vi "Intialise or refresh queue.vi"(2 "When did you stick it in?":dbl, 3 "Cell Settings Array":T3=[{"Measure?"=TRUE, "Area (cm^2)"=0.0, "Cell Label"="", "Cell Description"="", "Time between scans (s)"=0.0, "Cell Position"=1, "Scan settings in queue"=0, "Sample holder"=4.0, "User name"=""}, {"Measure?"=TRUE, "Area (cm^2)"=0.0, "Cell Label"="", "Cell Description"="", "Time between scans (s)"=0.0, "Cell Position"=2, "Scan settings in queue"=0, "Sample holder"=4.0, "User name"=""}, {"Measure?"=TRUE, "Area (cm^2)"=0.0, "Cell Label"="", "Cell Description"="", "Time between scans (s)"=0.0, "Cell Position"=3, "Scan settings in queue"=0, "Sample holder"=4.0, "User name"=""}, {"Measure?"=TRUE, "Area (cm^2)"=0.0, "Cell Label"="", "Cell Description"="", "Time between scans (s)"=0.0, "Cell Position"=4, "Scan settings in queue"=0, "Sample holder"=4.0, "User name"=""}, {"Measure?"=TRUE, "Area (cm^2)"=0.0, "Cell Label"="", "Cell Description"="", "Time between scans (s)"=0.0, "Cell Position"=5, "Scan settings in queue"=0, "Sample holder"=4.0, "User name"=""}, {"Measure?"=TRUE, "Area (cm^2)"=0.0, "Cell Label"="", "Cell Description"="", "Time between scans (s)"=0.0, "Cell Position"=6, "Scan settings in queue"=0, "Sample holder"=4.0, "User name"=""}, {"Measure?"=TRUE, "Area (cm^2)"=0.0, "Cell Label"="", "Cell Description"="", "Time between scans (s)"=0.0, "Cell Position"=7, "Scan settings in queue"=0, "Sample holder"=4.0, "User name"=""}, {"Measure?"=TRUE, "Area (cm^2)"=0.0, "Cell Label"="", "Cell Description"="", "Time between scans (s)"=0.0, "Cell Position"=8, "Scan settings in queue"=0, "Sample holder"=4.0, "User name"=""}, {"Measure?"=TRUE, "Area (cm^2)"=0.0, "Cell Label"="", "Cell Description"="", "Time between scans (s)"=0.0, "Cell Position"=9, "Scan settings in queue"=0, "Sample holder"=4.0, "User name"=""}, {"Measure?"=TRUE, "Area (cm^2)"=0.0, "Cell Label"="", "Cell Description"="", "Time between scans (s)"=0.0, "Cell Position"=10, "Scan settings in queue"=0, "Sample holder"=4.0, "User name"=""}, {"Measure?"=TRUE, "Area (cm^2)"=0.0, "Cell Label"="", "Cell Description"="", "Time between scans (s)"=0.0, "Cell Position"=11, "Scan settings in queue"=0, "Sample holder"=4.0, "User name"=""}, {"Measure?"=TRUE, "Area (cm^2)"=0.0, "Cell Label"="", "Cell Description"="", "Time between scans (s)"=0.0, "Cell Position"=12, "Scan settings in queue"=0, "Sample holder"=4.0, "User name"=""}, {"Measure?"=TRUE, "Area (cm^2)"=0.0, "Cell Label"="", "Cell Description"="", "Time between scans (s)"=0.0, "Cell Position"=13, "Scan settings in queue"=0, "Sample holder"=4.0, "User name"=""}, {"Measure?"=TRUE, "Area (cm^2)"=0.0, "Cell Label"="", "Cell Description"="", "Time between scans (s)"=0.0, "Cell Position"=14, "Scan settings in queue"=0, "Sample holder"=4.0, "User name"=""}, {"Measure?"=TRUE, "Area (cm^2)"=0.0, "Cell Label"="", "Cell Description"="", "Time between scans (s)"=0.0, "Cell Position"=15, "Scan settings in queue"=0, "Sample holder"=4.0, "User name"=""}, {"Measure?"=TRUE, "Area (cm^2)"=0.0, "Cell Label"="", "Cell Description"="", "Time between scans (s)"=0.0, "Cell Position"=16, "Scan settings in queue"=0, "Sample holder"=4.0, "User name"=""}] {"Scan settings in queue" items=["Standard"]}, 4 "Queue in":T1 {"Scan settings in queue" items=["Regular", "Inverted", "MartinaSettings"]; "Time of the last scan (s)" format="%<%H:%M:%S>t"; "When did you stick it in?" format="%<%H:%M:%S>t"; "Time to next scan (s)" format="%<%H:%M:%S>t"; "Time in rig (s)" format="%<%H:%M:%S>t"}) -> (0 "Queue out":T1 {"Scan settings in queue" items=["Regular", "Inverted", "MartinaSettings"]; "Time of the last scan (s)" format="%<%H:%M:%S>t"; "When did you stick it in?" format="%<%H:%M:%S>t"; "Time to next scan (s)" format="%<%H:%M:%S>t"; "Time in rig (s)" format="%<%H:%M:%S>t"})   [LabVIEW 2011]
uses:
  Typedefs/Cell details array.ctl
  Typedefs/Cell details cluster.ctl
  Typedefs/Queue.ctl
  Typedefs/Queue cluster.ctl
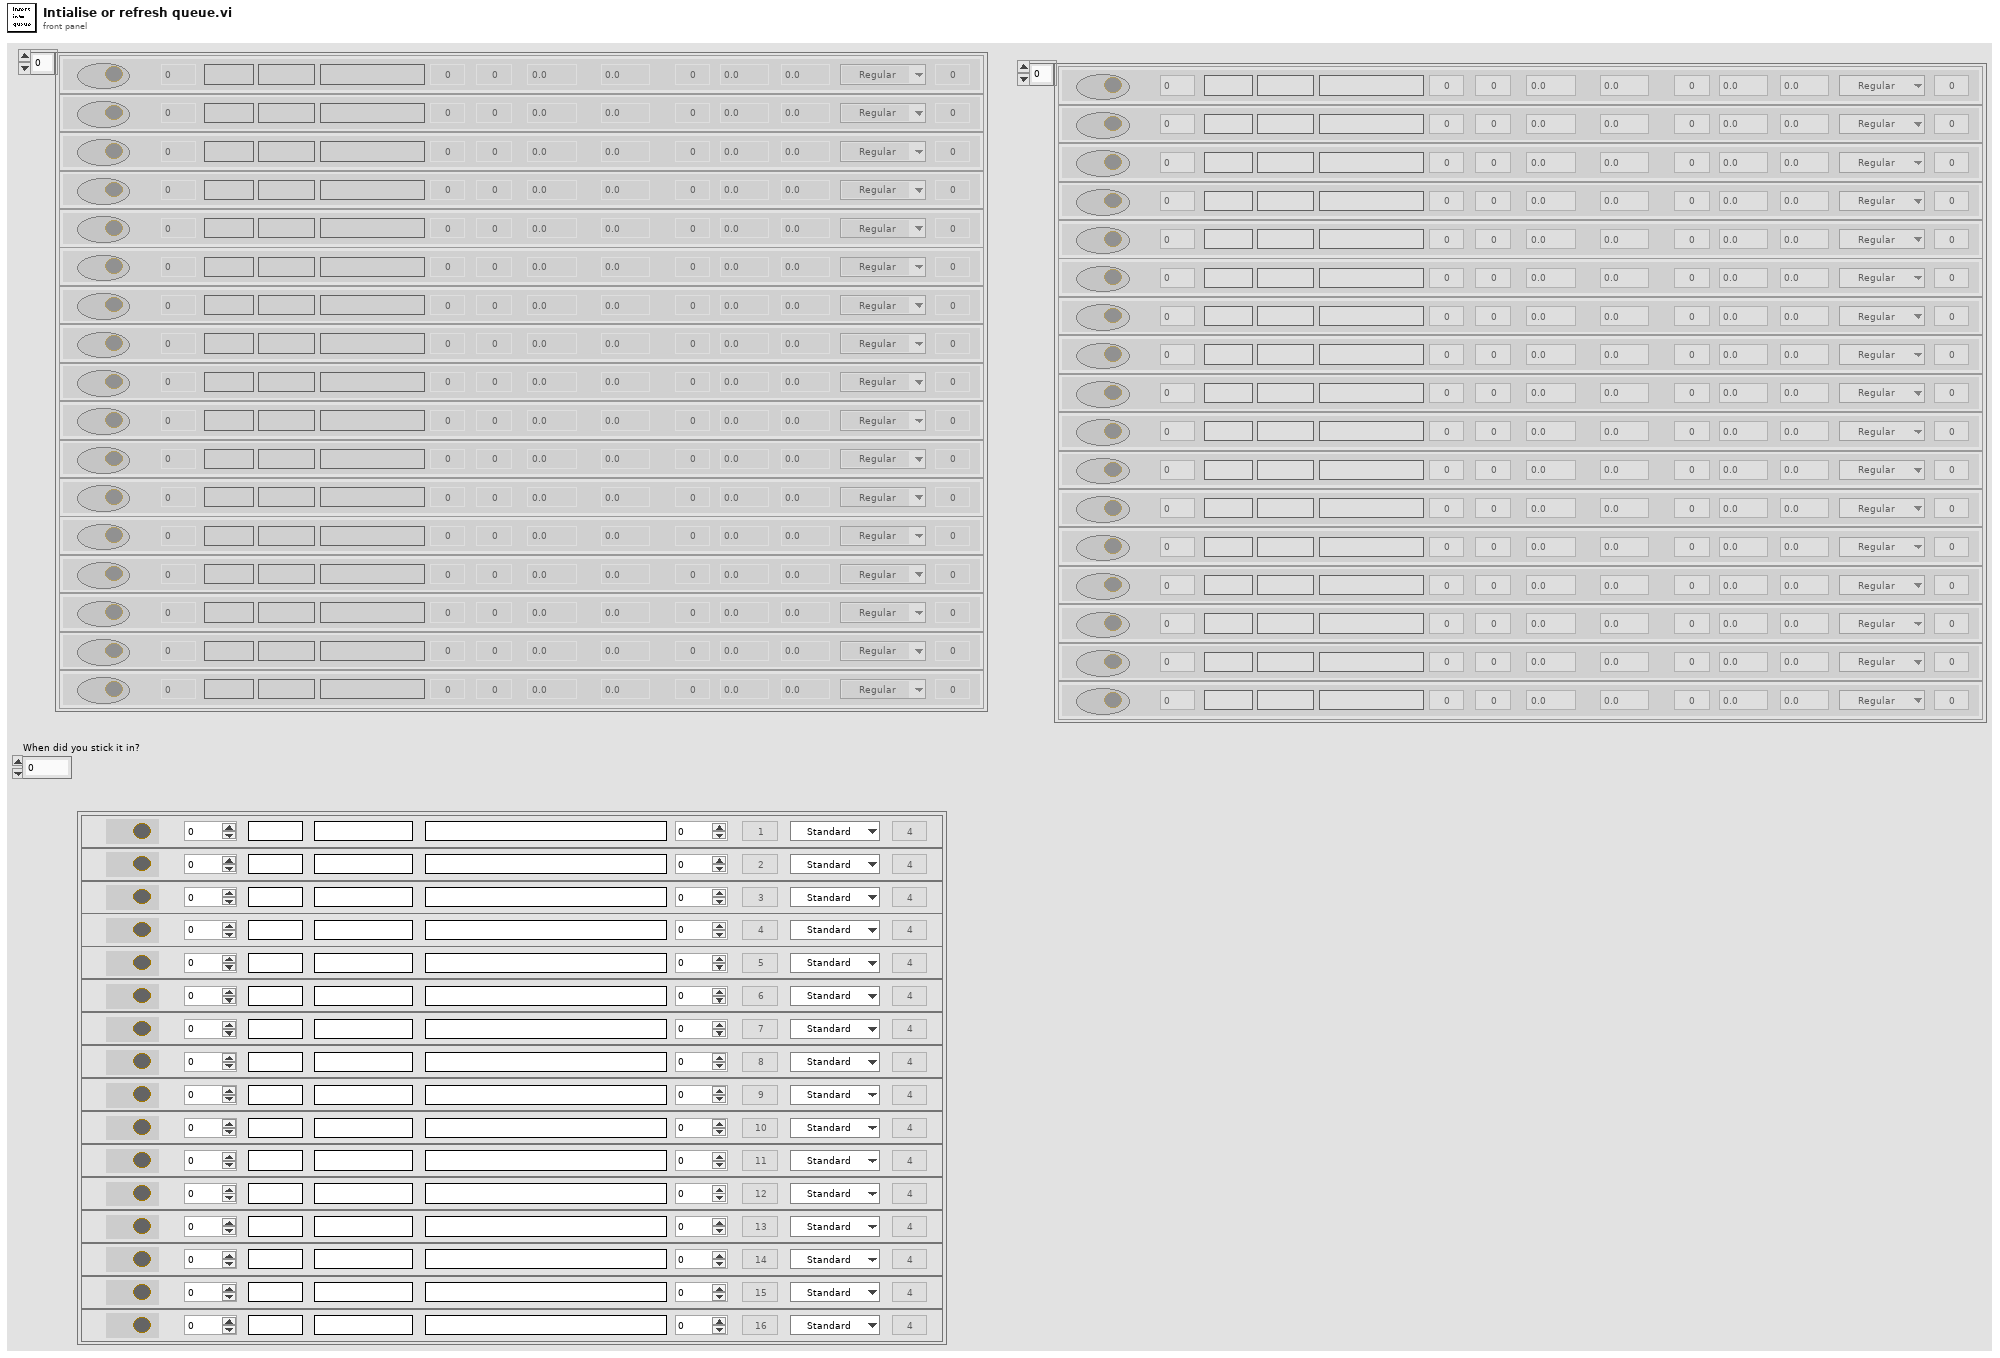
[diagram p1: front panel]
types:
  T1 = typedef "Queue.ctl" = T2[]
  T2 = typedef "Queue cluster.ctl" = cluster{"Measure?":bool, "Area (cm^2)":dbl, "Cell Label":string, "Cell Description":string, "Cell Position":i32, "Time in rig (s)":dbl, "Time to next scan (s)":dbl, "Scan number":dbl, "When did you stick it in?":dbl, "Time between scans (s)":dbl, "Time of the last scan (s)":dbl, "Scan settings in queue":u16, "Sample Holder":dbl, "User Name":string}
  T3 = typedef "Cell details array.ctl" = T4[]
  T4 = typedef "Cell details cluster.ctl" = cluster{"Measure?":bool, "Area (cm^2)":dbl, "Cell Label":string, "Cell Description":string, "Time between scans (s)":dbl, "Cell Position":i32, "Scan settings in queue":u16, "Sample holder":dbl, "User name":string}
  T5 = cluster{"Measure?":bool, "Area (cm^2)":dbl, "Cell Label":string, "Cell Description":string, "Cell Position":i32, "Time in rig (h)":dbl, "Time to next scan (min)":dbl, "Scan number":dbl, "When did you stick it in?":dbl, "Time between scans (min)":dbl, "Time of the last scan(min)":dbl, "Scan settings in queue":u16, "Sample Holder":dbl, "User Name":string}[]
  T6 = cluster{"Measure?":bool, "Area (cm^2)":dbl, "Cell Label":string, "Cell Description":string, "Cell Position":i32, "Time in rig (s)":dbl, "Time to next scan (s)":dbl, "Scan number":dbl, "When did you stick it in?":dbl, "Time between scans (s)":dbl, "Time of the last scan (s)":dbl, "Scan settings in queue":u16, "Sample Holder":dbl, "User Name":string}
  T7 = cluster{"Measure?":bool, "Area (cm^2)":dbl, "Cell Label":string, "Cell Description":string, "Cell Position":i32, "Time in rig (h)":dbl, "Time to next scan (min)":dbl, "Scan number":dbl, "When did you stick it in?":dbl, "Time between scans (min)":dbl, "Time of the last scan(min)":dbl, "Scan settings in queue":u16, "Sample Holder":dbl, "User Name":string}
  T8 = cluster{"Measure?":bool, "Area (cm^2)":dbl, "Cell Label":string, "Cell Description":string, "Cell Position":i32, "Time in rig (s)":dbl, "Time to next scan (s)":dbl, "Scan number":dbl, "When did you stick it in?":dbl, "Time between scans (s)":dbl, "Time of the last scan (s)":dbl, "Scan settings in queue":u16, "Sample Holder":dbl, "User Name":string}[]
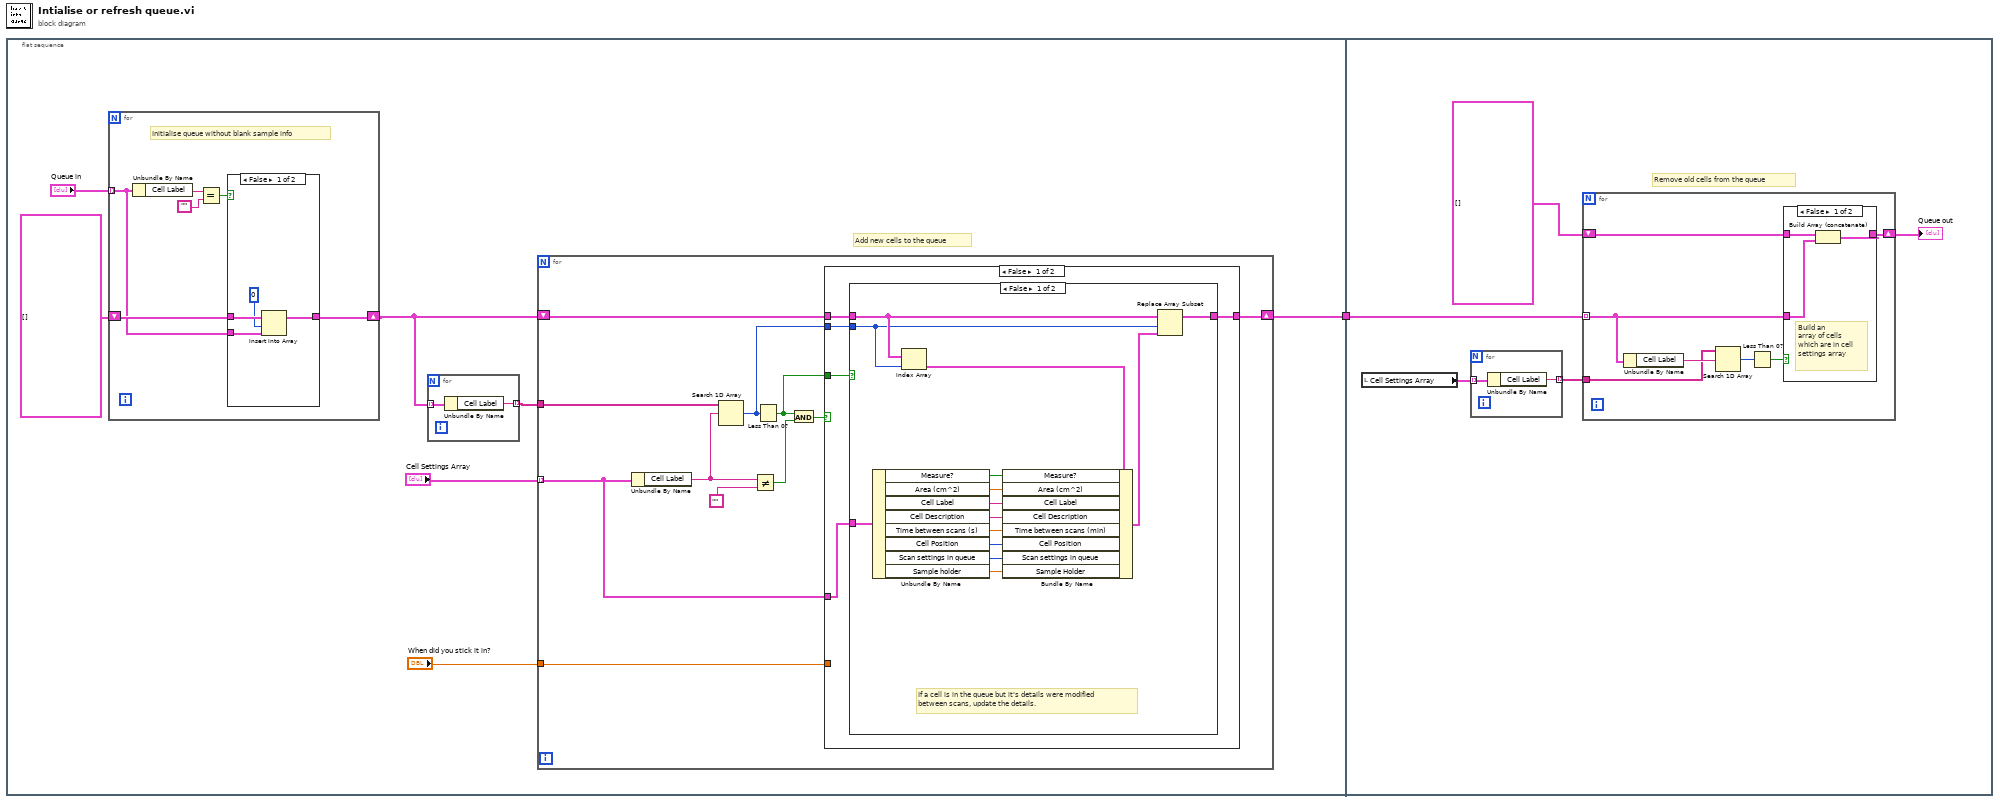
[diagram p0: block diagram]
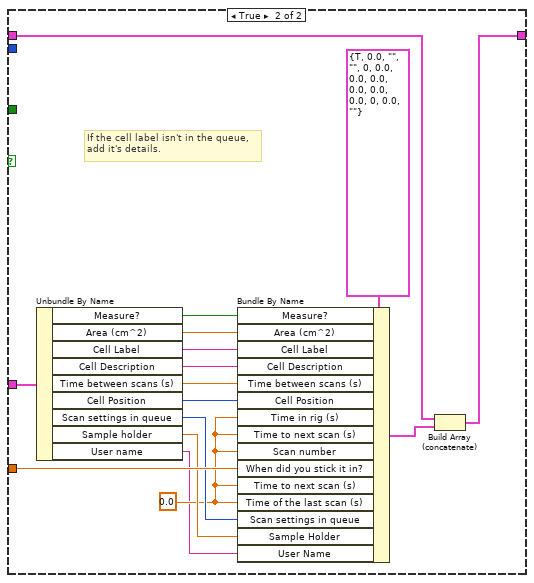
[diagram p4: hidden frame]
diagram:
  n1 = flat-sequence {
    tunnel: [w3] -> w1
    tunnel: w1 -> [w69]
    frame #0 {
      # "Add new cells to the queue"
      n2 = for {
        tunnel: "Queue in" -> [w10] mode=indexing
        shift-right: [w9] -> w2
        shift-left: T5 [] -> [w11]
        # "Initialise queue without blank sample info"
        n3 = Unbundle By Name(w10) -> ("Cell Label"=w14:string)
        n4 = Equal?(x=w14, y="") -> (x = y?=w12:bool)
        n5 = case shown="False" w12 {
          tunnel: w11 -> [w18 w19]
          tunnel: w10 -> [w16 _]
          tunnel: [w15 w19] -> w9
          frame False {
            n6 = Insert Into Array(array=w18, index=0, new element=w16) -> (w15:T5)
          }
          frame True {
          }
        }
      }
      n7 = for {
        tunnel: w2 -> [w21] mode=indexing
        tunnel: [w20] -> w7 mode=indexing
        n8 = Unbundle By Name(w21) -> ("Cell Label"=w20:string)
      }
      n9 = for {
        tunnel: "Cell Settings Array" -> [w30] mode=indexing
        tunnel: "When did you stick it in?" -> [w31]
        tunnel: w7 -> [w32]
        shift-right: [w28] -> w3
        shift-left: w2 -> [w29]
        n10 = Unbundle By Name(w30) -> ("Cell Label"=w27:string)
        n11 = Search 1D Array(1D array=w32, element=w27) -> (index of element=w22:i32)  [unwired: 1 in]
        n12 = Not Equal?(x=w27, y="") -> (x != y?=w25:bool)
        n13 = Less Than 0?(x=w22) -> (x < 0?=w23:bool)
        n14 = And(x=w23, y=w25) -> (x .and. y?=w24:bool)
        n15 = case shown="False" w24 {
          tunnel: w31 -> [_ w67]
          tunnel: w30 -> [w34 w66]
          tunnel: w29 -> [w36 w57]
          tunnel: [w33 w56] -> w28
          tunnel: w23 -> [w37 _]
          tunnel: w22 -> [w35 _]
          frame False {
            n16 = case shown="False" w37 {
              tunnel: w36 -> [w41 w52]
              tunnel: w35 -> [w39 _]
              tunnel: w34 -> [w51 _]
              tunnel: [w40 w52] -> w33
              frame False {
                # "If a cell is in the queue but it's details were modified\nbetween scans, update the details."
                n17 = Unbundle By Name(w51) -> ("Measure?"=w49:bool, "Area (cm^2)"=w48:dbl, "Cell Label"=w47:string, "Cell Description"=w46:string, "Time between scans (s)"=w45:dbl, "Cell Position"=w44:i32, "Scan settings in queue"=w43:u16, "Sample holder"=w42:dbl)
                n18 = Index Array(array=w41, index=w39) -> (element=w50:T7)
                n19 = Bundle By Name(cluster=w50, "Measure?"=w49, "Area (cm^2)"=w48, "Cell Label"=w47, "Cell Description"=w46, "Time between scans (min)"=w45, "Cell Position"=w44, "Scan settings in queue"=w43, "Sample Holder"=w42) -> (w38:T7)
                n20 = Replace Array Subset(array=w41, new element=w38, index=w39) -> (w40:T5)
              }
              frame True {
                # "If a cell isn't in the queue there is nothing to update"
              }
            }
          }
          frame True {
            w54 = 0.0 ("Time of the last scan (min)")
            # "If the cell label isn't in the queue,\nadd it's details."
            n21 = Unbundle By Name(w66) -> ("Measure?"=w65:bool, "Area (cm^2)"=w64:dbl, "Cell Label"=w63:string, "Cell Description"=w62:string, "Time between scans (s)"=w61:dbl, "Cell Position"=w60:i32, "Scan settings in queue"=w59:u16, "Sample holder"=w55:dbl, "User name"=w53:string)
            n22 = Bundle By Name(cluster=T6 {"Measure?"=TRUE, "Area (cm^2)"=0.0, "Cell Label"="", "Cell Description"="", "Cell Position"=0, "Time in rig (s)"=0.0, "Time to next scan (s)"=0.0, "Scan number"=0.0, "When did you stick it in?"=0.0, "Time between scans (s)"=0.0, "Time of the last scan (s)"=0.0, "Scan settings in queue"=0, "Sample Holder"=0.0, "User Name"=""} ("Cluster"), "Measure?"=w65, "Area (cm^2)"=w64, "Cell Label"=w63, "Cell Description"=w62, "Time between scans (s)"=w61, "Cell Position"=w60, "Time in rig (s)"=w54, "Time to next scan (s)"=w54, "Scan number"=w54, "When did you stick it in?"=w67, "Time to next scan (s)"=w54, "Time of the last scan (s)"=w54, "Scan settings in queue"=w59, "Sample Holder"=w55, "User Name"=w53) -> (w58:T6)
            n23 = Build Array (concatenate)(w57, w58) -> (w56:T8)
          }
        }
      }
    }
    frame #1 {
      # "Remove old cells from the queue"
      n24 = local read "Cell Settings Array"() -> (w72:T3)
      n25 = for {
        tunnel: w72 -> [w75] mode=indexing
        tunnel: [w74] -> w70 mode=indexing
        n26 = Unbundle By Name(w75) -> ("Cell Label"=w74:string)
      }
      n27 = for {
        tunnel: w70 -> [w81]
        tunnel: w69 -> [w77] mode=indexing
        shift-right: [w76] -> w73
        shift-left: T5 [] -> [w79]
        n28 = Unbundle By Name(w77) -> ("Cell Label"=w82:string)
        n29 = Search 1D Array(1D array=w81, element=w82) -> (index of element=w80:i32)  [unwired: 1 in]
        n30 = Less Than 0?(x=w80) -> (x < 0?=w78:bool)
        n31 = case shown="False" w78 {
          tunnel: w79 -> [w85 w86]
          tunnel: w77 -> [w84 _]
          tunnel: [w83 w86] -> w76
          frame False {
            # "Build an\narray of cells\nwhich are in cell\nsettings array"
            n32 = Build Array (concatenate)(w85, w84) -> (w83:T5)
          }
          frame True {
          }
        }
      }
      "Queue out" <- w73
    }
  }
